vi "E710_WaveGenerator_Sample_Program.vi"(0 "System no.":i32=1 min=1 step=1, 2 "Affected axis":string, 3 "Choice":bool[](array[boolean])=[FALSE, FALSE, FALSE, FALSE, FALSE, FALSE, FALSE, FALSE, FALSE, FALSE, FALSE, FALSE, FALSE, FALSE, FALSE, FALSE, FALSE, FALSE, FALSE, FALSE, FALSE, FALSE, FALSE, FALSE, FALSE, FALSE, FALSE, FALSE, FALSE, FALSE, FALSE, FALSE], 4 "DDL":bool, 5 "error in":errorcluster, 6 "Xo (Start)":i32, 7 "SIN_P Parameters":cluster{"C":dbl, "A":dbl, "O":dbl}={"C"=200.0, "A"=50.0, "O"=0.0} {"O" format="%.6f"; "A" format="%.6f"; "C" format="%.6f"}, 8 "N (Length)":i32=500 min=0 max=1000 step=1, 9 "Append? (&)":bool, 10 "Xo (Start)":i32, 11 "RAMP Parameters":cluster{"C":dbl, "J":dbl, "A":dbl, "O":dbl}={"C"=200.0, "J"=0.0, "A"=20.0, "O"=0.0} {"O" format="%.6f"; "A" format="%.6f"; "J" format="%.6f"; "C" format="%.6f"}, 12 "N (Length)":i32=500 min=0 max=1000 step=1, 13 "Append? (&)":bool) -> (14 "Waveform":dbl[][](graph) caption="Graph showing the commanded (green) and measured (white) waveform and the position error (red).", 19 "Error out":errorcluster)   [LabVIEW 2011]
doc: "This VI demonstrates how to use the wave generator command VI's of the E-710. It first moves the affected axis to a start position of zero. Then it runs in a loop, giving the user the options to write sine wave curve segments or ramps into the E-710 wave buffer. Wave storage data points are limited to 1000 points to keep transfer times low. The segment length of one waveform - which normally defines the frequency - is predefined as 500 points in this example. Depending on the value of Append? (&), either the old buffer data is overwritten or the new wave will be appended to memory. Please take into account that you can append at most two waveforms since buffer size is limited to 1000 points as mentioned above. \n\nAdjust the following controls to modify the shape of the waveforms.\nN (Length): Waveform (i.e. the points to be modified) goes from 0 to Length. Datapoints from Length to 500 are filled with zeros.\nXo (Start): Position where the first point of the waveform is located. \nC: Center point of the wave. If C = Length/2 then the wave is symmetrical.\nA: Amplitude of the waveform. F(x) = A*sin(x) + O\nO: Offset of the waveform. F(x) = A*sin(x) + O\nJ: Jerk. Means curvature in the transition to or from standstill.\n\nYou have to stop generator output prior to restarting it with a different parameter set. Otherwise you get a Hidden error. The Start Gen. and Stop Gen. buttons will enable or disable the wave generator output by sending \"WGO 0\" or \"WGO 1\" for the affected axis. The red Stop button stops the wave generator output on the specified axis and finishes the loop. \n\nPlease respect the delays that occur while the controller is processing your commands. This is indicated by the Writing... indicator. \n\nIn case of an error a button \"Clear Error\" will appear and the control buttons above will be disabled. Pressing this button will clear the error status and enable the control buttons again.\n\nWith DDL ON you can achieve significantly better position accuracy. Compare the target (green), response (white) and error (red) signals on the graph. Since this is a very sensitive mechanism we recommend starting with low amplitudes and adjusting the parameters with caution. The DDL button works only if the controller supports DDL. Contact PI for information on activation of DDL support.\nRun E710_Configuration_Setup prior to running this VI. \n\nValid for: E-710"
panel:
  out "DDL":bool
  in  "Clear Error":bool
  out "Busy?":bool
  out "Hidden error":bool
  in  "Stop wave generator \noutput":bool
  # "E-710 wave generator sample program"
  # "This VI demonstrates how to use the wave generator command VIs of the E-710. It first moves the affected axis to a start position of zero. Then it runs in a \nloop, giving the user the options to write sine wave curve segments or ramps into the E-710 wave buffer. Wave storage data points are limited to 1000 points\nto keep transfer times low. The segment length of one waveform is predefined as 500 points in this example. Depending on the value of Append? (&), either\nthe old buffer data is overwritten or the new wave will be appended to memory. You have to stop generator output prior to restarting it with a different\nparameter set. The Start Gen. and Stop Gen. buttons will enable or disable the wave generator output by sending \"WGO 0\" or \"WGO 1\" for the affected axis. \nIf DDL is enabled \"WGO 65\" will be sent respectively. The red Stop button stops the wave generator output on the specified axis and finishes the loop. \nPlease respect the delays that occur while the controller is processing your commands. This is indicated by the \"Busy?\" indicator. See manual for further details. \nRun E710_Configuration_Setup prior to running this VI."
  # "Sine Parameters:"
  # "Ramp Parameters:"
  # "Write Sine"
  # "Write Ramp"
  # "DDL state"
  # "Start Gen"
  # "Stop\nwave\ngenerator\noutput"
  # "Stop Gen"
  # "Read Buffer"
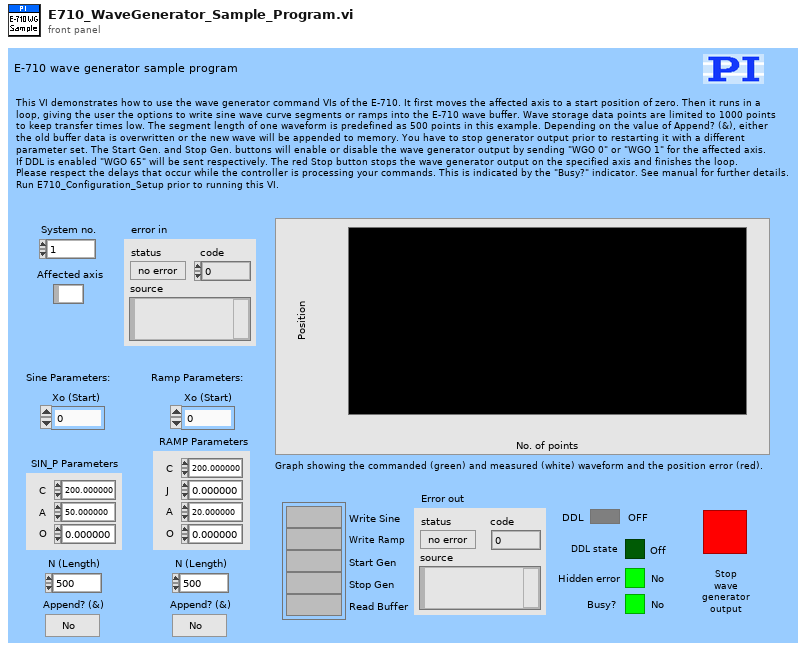
[diagram p1: front panel]
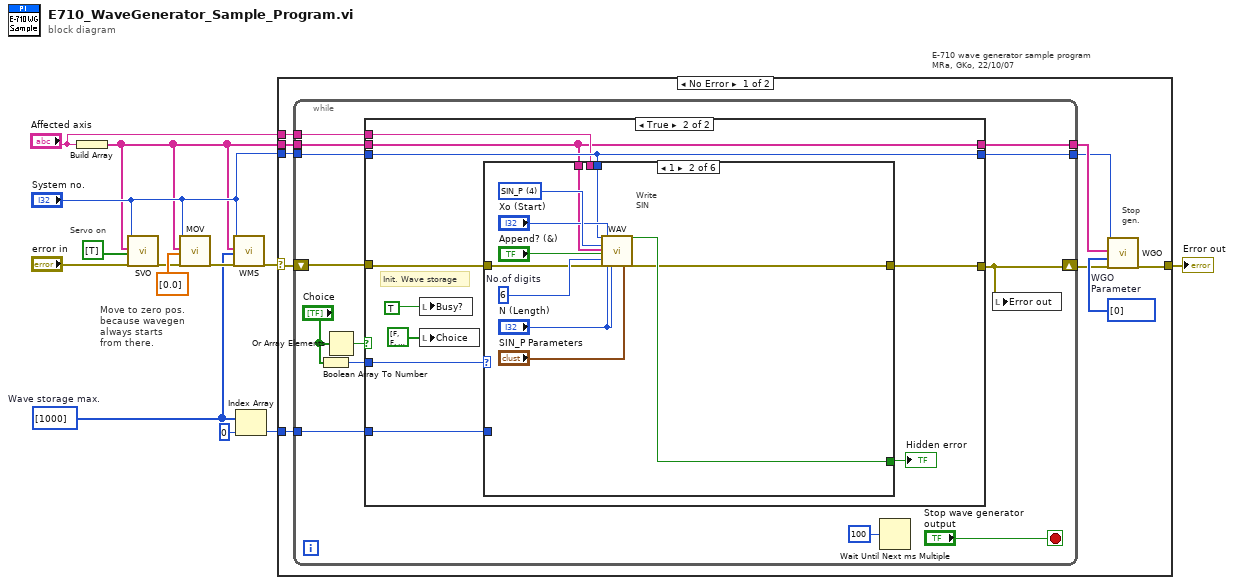
[diagram p0: block diagram]
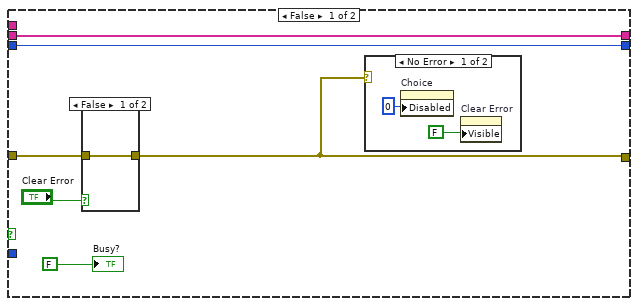
[diagram p2: hidden frame]
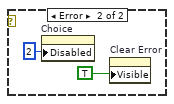
[diagram p3: hidden frame]
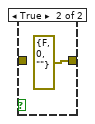
[diagram p4: hidden frame]
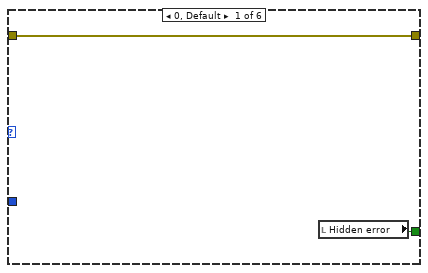
[diagram p5: hidden frame]
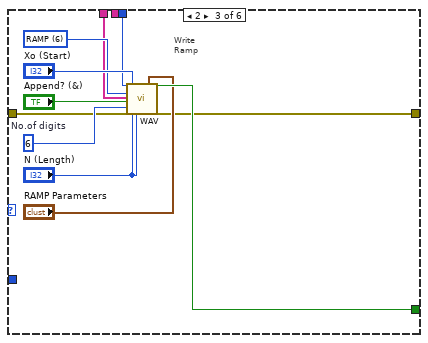
[diagram p6: hidden frame]
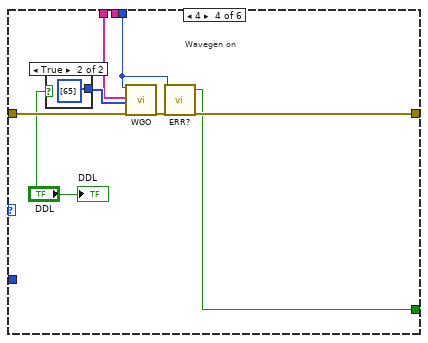
[diagram p7: hidden frame]
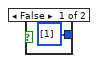
[diagram p8: hidden frame]
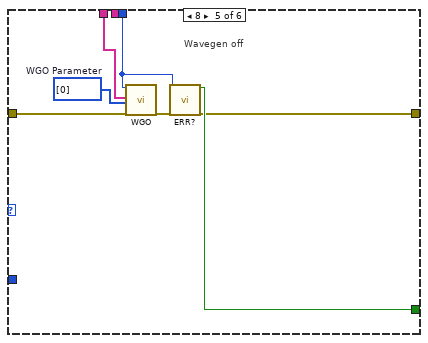
[diagram p9: hidden frame]
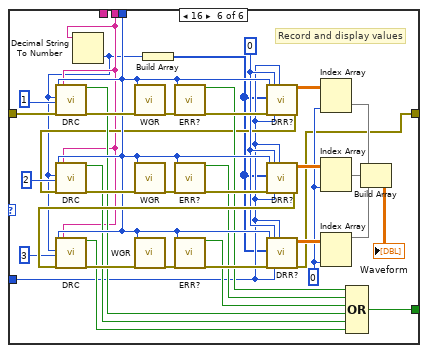
[diagram p10: hidden frame]
diagram:
  w3 = i32[] [1000]  # Wave storage max.
  # "Servo on"
  # "Move to zero pos.\nbecause wavegen\nalways starts \nfrom there."
  # "E-710 wave generator sample program\nMRa, GKo, 22/10/07"
  n1 = Build Array("Affected axis") -> (w6:string[])
  n2 = call "SVO.vi"("System no."="System no.", "Axes to command"=w6, "Servo mode"=bool[] [TRUE]) -> ()  [unwired: 2 in, 15 out]
  n3 = call "MOV.vi"("System no."="System no.", "Axes to move"=w6, "Position values"=dbl[] [0.0], "error in"="error in") -> ("error out"=w9:errorcluster)  [unwired: 1 in, 14 out]
  n4 = call "WMS.vi"("System no."="System no.", "Axes to set"=w6, "Wave storage max."=w3, "error in"=w9) -> ("error out"=w5:errorcluster)  [unwired: 1 in, 14 out]
  n5 = Index Array(array=w3, index=0 ("Index")) -> (element=w4:i32)
  n6 = case shown="No Error" w5 {
    selector: w5 -> [w15 w136]
    tunnel: w6 -> [w22 _]
    tunnel: "System no." -> [w21 _]
    tunnel: [w20 w136] -> w10
    tunnel: w4 -> [w14 _]
    tunnel: "Affected axis" -> [w13 _]
    frame No Error {
      w19 = i32[] [0]  # WGO  Parameter
      # "Stop\ngen."
      n7 = while {
        tunnel: w13 -> [w23]
        tunnel: w14 -> [w24]
        shift-left: w15 -> [w26]
        shift-right: [w25] -> w16
        tunnel: [w27] -> w17
        tunnel: [w29] -> w18
        tunnel: w21 -> [w28]
        tunnel: w22 -> [w30]
        stop <- "Stop wave generator \noutput" stop-if-true
        n8 = Boolean Array To Number(Boolean array="Choice") -> (number=w33:u32)
        n9 = Or Array Elements(Boolean array="Choice") -> (logical OR=w32:bool)
        n10 = case shown="True" w32 {
          tunnel: [w36 w53] -> w25
          tunnel: w33 -> [_ w55]
          tunnel: w28 -> [w40 w52]
          tunnel: w30 -> [w39 w48]
          tunnel: [w39 w48] -> w29
          tunnel: [w40 w52] -> w27
          tunnel: w26 -> [w38 w54]
          tunnel: w24 -> [_ w50]
          tunnel: w23 -> [_ w49]
          frame False {
            n11 = case shown="False" "Clear Error" {
              tunnel: w38 -> [w46 _]
              tunnel: [w46 errorcluster {"status"=FALSE, "code"=0, "source"=""} ("error IO")] -> w36
              frame False {
              }
              frame True {
              }
            }
            n12 = case shown="No Error" w36 {
              frame No Error {
                n13 = property on="Choice" class="Arr (strict)"("Disabled"=u8 0) -> ()  [unwired: 2 in, 2 out]
                n14 = property on="Clear Error" class="Bool"("Visible"=FALSE) -> ()  [unwired: 2 in, 2 out]
              }
              frame Error {
                n15 = property on="Choice" class="Arr (strict)"("Disabled"=u8 2) -> ()  [unwired: 2 in, 2 out]
                n16 = property on="Clear Error" class="Bool"("Visible"=TRUE) -> ()  [unwired: 2 in, 2 out]
              }
            }
            "Busy?" <- FALSE
          }
          frame True {
            # "Init. Wave storage"
            n17 = local write "Busy?"(TRUE) -> ()
            n18 = local write "Choice"(bool[] [FALSE, FALSE, FALSE, FALSE, FALSE, FALSE, FALSE, FALSE, FALSE, FALSE, FALSE, FALSE, FALSE, FALSE, FALSE, FALSE, FALSE, FALSE, FALSE, FALSE, FALSE, FALSE, FALSE, FALSE, FALSE, FALSE, FALSE, FALSE, FALSE, FALSE, FALSE, FALSE] ("Choice")) -> ()
            n19 = case shown="1" w55 {
              tunnel: [w59 w65 w77 w85 w96 w131] -> w51
              tunnel: [w58 w64 w75 w87 w94 w103] -> w53
              tunnel: w54 -> [w58 w63 w74 w88 w97 w134]
              tunnel: w49 -> [_ _ _ _ _ w101]
              tunnel: w52 -> [_ w62 w73 w83 w93 w123]
              tunnel: w50 -> [_ _ _ _ _ w102]
              tunnel: w48 -> [_ w61 w72 w82 w92 _]
              frame 0, Default {
                n20 = local read "Hidden error"() -> (w59:bool)
              }
              frame 1 {
                w67 = i16 6  # No.of digits
                w70 = u16 4 items=["SIN", "POL", "TAN", "PNT", "SIN_P", "LIN", "RAMP"] ("Waveform")
                # "Write\nSIN"
                n21 = call "WAV.vi"("System no."=w62, "Waveform"=w70, "Affected axes"=w61, "Append? (&)"="Append? (&)", "No.of digits"=w67, "error in"=w63, "Xo"="Xo (Start)", "N"="N (Length)", "Segment length"="N (Length)", "SIN_P Parameters"="SIN_P Parameters") -> ("Controller error"=w65:bool, "error out"=w64:errorcluster)  [unwired: 8 in, 8 out]
              }
              frame 2 {
                w78 = u16 6 items=["SIN", "POL", "TAN", "PNT", "SIN_P", "LIN", "RAMP"] ("Waveform")
                w80 = i16 6  # No.of digits
                # "Write\nRamp"
                n22 = call "WAV.vi"("System no."=w73, "Waveform"=w78, "Affected axes"=w72, "Append? (&)"="Append? (&)", "No.of digits"=w80, "error in"=w74, "Xo"="Xo (Start)", "N"="N (Length)", "Segment length"="N (Length)", "RAMP Parameters"="RAMP Parameters") -> ("Controller error"=w77:bool, "error out"=w75:errorcluster)  [unwired: 8 in, 8 out]
              }
              frame 4 {
                # "Wavegen on"
                n23 = case shown="True" "DDL" {
                  tunnel: [i32[] [1] ("WGO Parameter") i32[] [65] ("WGO Parameter")] -> w89
                  frame False {
                  }
                  frame True {
                  }
                }
                n24 = call "WGO.vi"("System no."=w83, "Affected axes"=w82, "WGO Parameter"=w89, "error in"=w88) -> ("error out"=w86:errorcluster)  [unwired: 15 out]
                n25 = call "ERR?.vi"("System no."=w83, "error in"=w86) -> ("Controller error"=w85:bool, "error out"=w87:errorcluster)  [unwired: 16 out]
                "DDL" <- "DDL"
              }
              frame 8 {
                w98 = i32[] [0]  # WGO Parameter
                # "Wavegen off"
                n26 = call "WGO.vi"("System no."=w93, "Affected axes"=w92, "WGO Parameter"=w98, "error in"=w97) -> ("error out"=w95:errorcluster)  [unwired: 15 out]
                n27 = call "ERR?.vi"("System no."=w93, "error in"=w95) -> ("Controller error"=w96:bool, "error out"=w94:errorcluster)  [unwired: 16 out]
              }
              frame 16 {
                w108 = 0 ("Disabled Index (col)")
                w122 = 0 ("Xo")
                # "Record and display values"
                n28 = Decimal String To Number(string=w101) -> (number=w99:i32)  [unwired: 3 out]
                n29 = call "DRC.vi"("System no."=w123, "Rec. table"=w99, "Rec. option"=1 ("Numeric"), "error in"=w134, "Source ID"=w101) -> ("Controller error"=w118:bool, "error out"=w133:errorcluster)  [unwired: 1 in, 12 out]
                n30 = call "WGR.vi"("System no."=w123, "error in"=w133) -> ("error out"=w135:errorcluster)  [unwired: 2 in, 15 out]
                n31 = Build Array(w99) -> (w100:i32[])
                n32 = call "ERR?.vi"("System no."=w123, "error in"=w135) -> ("Controller error"=w121:bool, "error out"=w132:errorcluster)  [unwired: 16 out]
                n33 = call "DRR?.vi"("System no."=w123, "Rec. table IDs"=w100, "error in"=w132, "Xo"=w122, "N"=w102, "Nmax"=w102) -> ("Data"=w109:dbl[][], "error out"=w104:errorcluster)  [unwired: 1 in, 11 out]
                n34 = call "DRC.vi"("System no."=w123, "Rec. table"=w99, "Rec. option"=2 ("Numeric"), "error in"=w104, "Source ID"=w101) -> ("Controller error"=w117:bool, "error out"=w129:errorcluster)  [unwired: 1 in, 12 out]
                n35 = call "WGR.vi"("System no."=w123, "error in"=w129) -> ("error out"=w128:errorcluster)  [unwired: 2 in, 15 out]
                n36 = call "ERR?.vi"("System no."=w123, "error in"=w128) -> ("Controller error"=w120:bool, "error out"=w130:errorcluster)  [unwired: 16 out]
                n37 = call "DRR?.vi"("System no."=w123, "Rec. table IDs"=w100, "error in"=w130, "Xo"=w122, "N"=w102, "Nmax"=w102) -> ("Data"=w111:dbl[][], "error out"=w127:errorcluster)  [unwired: 1 in, 11 out]
                n38 = call "DRC.vi"("System no."=w123, "Rec. table"=w99, "Rec. option"=3 ("Numeric"), "error in"=w127, "Source ID"=w101) -> ("Controller error"=w116:bool, "error out"=w125:errorcluster)  [unwired: 1 in, 12 out]
                n39 = call "WGR.vi"("System no."=w123, "error in"=w125) -> ("error out"=w126:errorcluster)  [unwired: 2 in, 15 out]
                n40 = call "ERR?.vi"("System no."=w123, "error in"=w126) -> ("Controller error"=w119:bool, "error out"=w124:errorcluster)  [unwired: 16 out]
                n41 = call "DRR?.vi"("System no."=w123, "Rec. table IDs"=w100, "error in"=w124, "Xo"=w122, "N"=w102, "Nmax"=w102) -> ("Data"=w110:dbl[][], "error out"=w103:errorcluster)  [unwired: 1 in, 11 out]
                n42 = Index Array(array=w109, index (col)=w108) -> (element=w106:dbl[])  [unwired: 1 in]
                n43 = Index Array(array=w111, index (col)=w108) -> (element=w107:dbl[])  [unwired: 1 in]
                n44 = Index Array(array=w110, index (col)=w108) -> (element=w105:dbl[])  [unwired: 1 in]
                n45 = Compound Arithmetic op=OR(w121, w120, w119, w118, w117, w116) -> (w131:bool)
                n46 = Build Array(w106, w107, w105) -> (→"Waveform":dbl[][])
              }
            }
            "Hidden error" <- w51
          }
        }
        n47 = Wait Until Next ms Multiple(millisecond multiple=u32 100) -> ()  [unwired: 1 out]
        n48 = local write "Error out"(w25) -> ()
      }
      n49 = call "WGO.vi"("System no."=w17, "Affected axes"=w18, "WGO Parameter"=w19, "error in"=w16) -> ("error out"=w20:errorcluster)  [unwired: 15 out]
    }
    frame Error {
    }
  }
  "Error out" <- w10
